vi "Pockels Cal_Get Wavelength header index.vi"(10 "Waveform":dbl, 11 "Loaded cal file":string[][](array[string])) -> (1 "Cal already exists for this wavelength?":bool, 2 "Index of \"Cal Wavelength\" header":i32)   [LabVIEW 2013]
panel:
  out "Indices of \"Cal Wavelength\" headers":i32[](array[numeric])
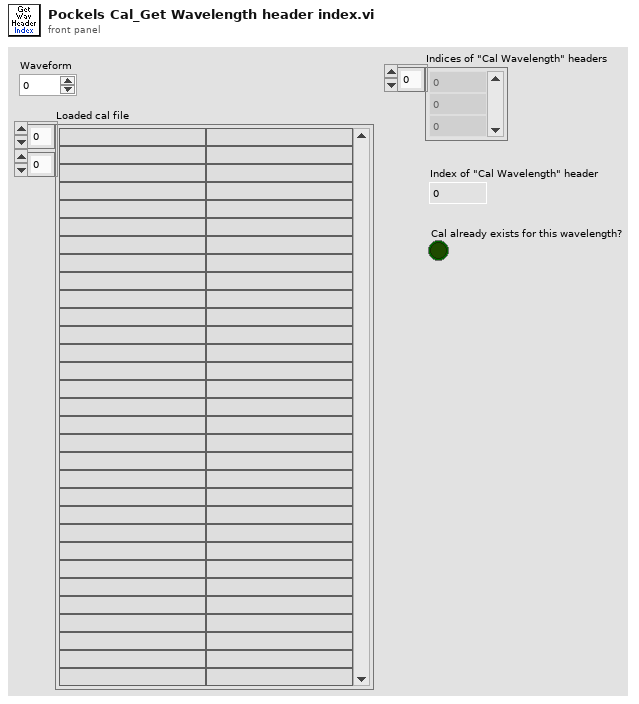
[diagram p1: front panel]
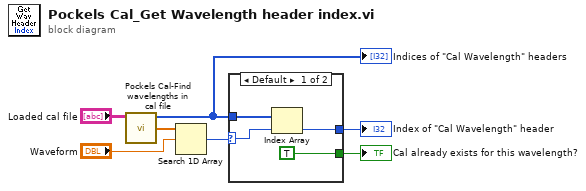
[diagram p0: block diagram]
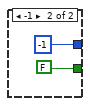
[diagram p2: hidden frame]
diagram:
  n1 = call "Pockels Cal-Find wavelengths in cal file.vi"("Loaded cal file"="Loaded cal file") -> ("Pockels cal'd wavelengths"=w5:dbl[], "Indices of Elements"=w2:i32[])  [unwired: 9 in]
  "Indices of \"Cal Wavelength\" headers" <- w2
  n2 = Search 1D Array(1D array=w5, element="Waveform") -> (index of element=w3:i32)  [unwired: 1 in]
  n3 = case shown="Default" w3 {
    selector: w3 -> [w9 _]
    tunnel: [TRUE FALSE] -> w4
    tunnel: w2 -> [w10 _]
    tunnel: [w8 -1 ("Numeric")] -> w1
    frame Default {
      n4 = Index Array(array=w10, index=w9) -> (element=w8:i32)
    }
    frame -1 {
    }
  }
  "Cal already exists for this wavelength?" <- w4
  "Index of \"Cal Wavelength\" header" <- w1
